vi "Read NET_HttpReponseMessage.vi"(8 "error in (no error)":errorcluster, 11 "HttpResponseMessage in":refnum<class "HttpResponseMessage.lvclass">) -> (0 "error out":errorcluster, 2 "NET_HttpReponseMessage":refnum<k24>, 3 "HttpResponseMessage out":refnum<class "HttpResponseMessage.lvclass">)   [LabVIEW 2018, in "LabVIEWHTTPClient_NET.lvlib" / "HttpResponseMessage.lvclass"]
uses:
  HttpResponseMessage.lvclass
  System.Net.Http
  HttpResponseMessage.lvclass/HttpResponseMessage.ctl
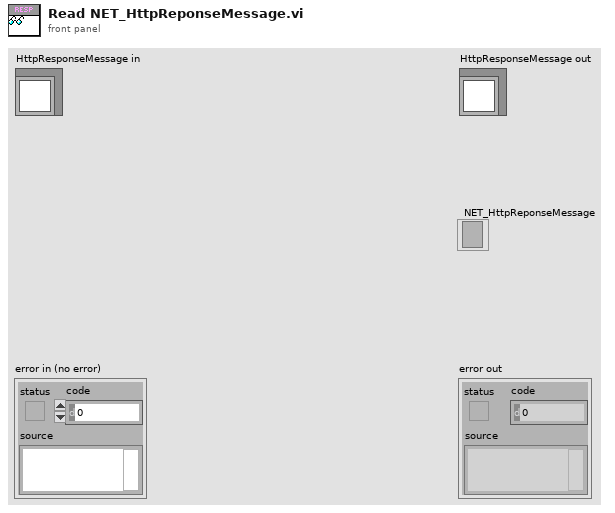
[diagram p1: front panel]
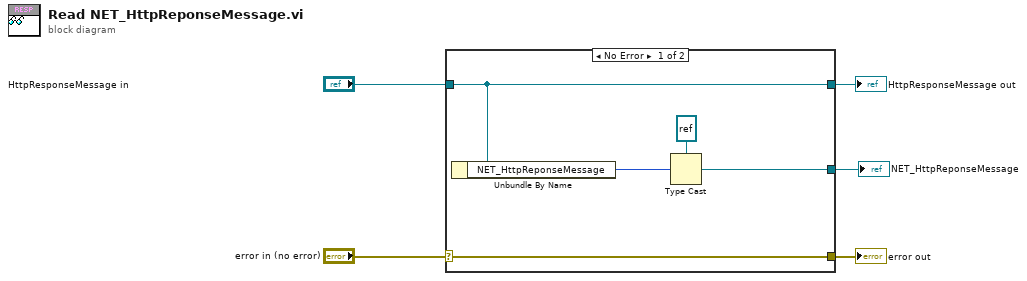
[diagram p0: block diagram]
diagram:
  n1 = case shown="No Error" "error in (no error)" {
    selector: "error in (no error)" -> [w10 w11]
    tunnel: [w10 w11] -> w4
    tunnel: [w9 w12] -> w2
    tunnel: "HttpResponseMessage in" -> [w9 w12]
    tunnel: [w7 _] -> w1
    frame No Error {
      n2 = Unbundle By Name(w9) -> ("NET_HttpReponseMessage"=w8:i64)
      n3 = Type Cast(type=refnum<k24> refnum ("NET_HttpReponseMessage"), x=w8) -> (*(type *) &x=w7:refnum<k24>)
    }
    frame Error {
    }
  }
  "error out" <- w4
  "HttpResponseMessage out" <- w2
  "NET_HttpReponseMessage" <- w1
